vi "Read AIP Status.vi"(8 "error in (no error)":errorcluster, 11 "AIP Status Response in":refnum<class "AIP Status Response.lvclass">) -> (0 "error out":errorcluster, 1 "AIP Depth Min":u8, 2 "AIP Status":T1, 3 "AIP Status Response out":refnum<class "AIP Status Response.lvclass">)   [LabVIEW 2015, in "RDS Child Messages.lvlib" / "AIP Status Response.lvclass"]
uses:
  AIP Status Response.lvclass
  RDS Instruments/AIP/AIP Status.ctl
  RDS Instruments/AIP/AIP States.ctl
  RDS Serial Handler/RDS Serial Frame.lvclass
  AIP Status Response.lvclass/AIP Status Response.ctl
  RDS Instruments/RDS Instrument Library.lvlib
panel:
  out "Raw Frame":refnum<class "RDS Serial Frame.lvclass">
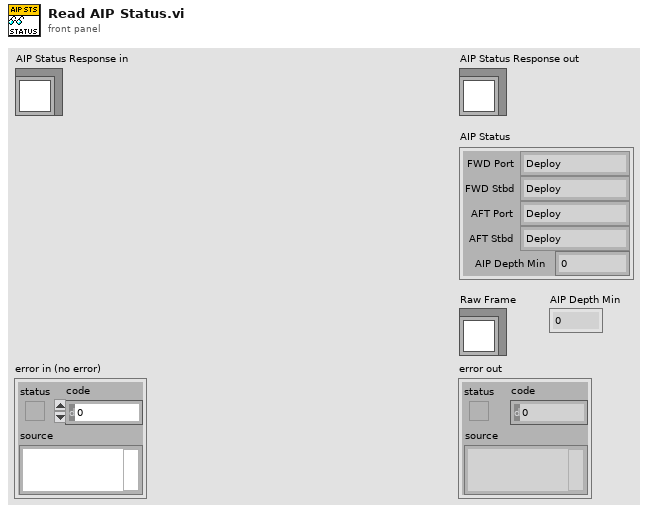
[diagram p1: front panel]
types:
  T1 = typedef "RDS Instrument Library.lvlib/AIP Status.ctl" = cluster{"FWD Port":T2, "FWD Stbd":T2, "AFT Port":T2, "AFT Stbd":T2, "AIP Depth Min":u8}
  T2 = typedef "RDS Instrument Library.lvlib/AIP States.ctl" = enum16{"Deploy", "Deploying", "Deployed", "Stow", "Stowing", "Stowed", "Fault", "brakeOnStow", "breakOnDeploy", "Stopped", "Stopping"}
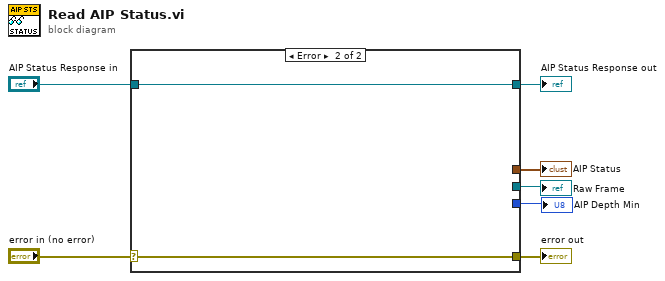
[diagram p0: block diagram]
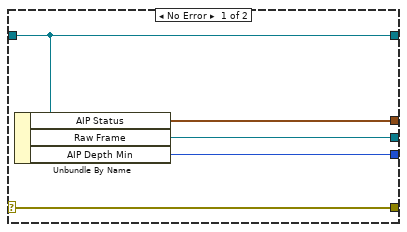
[diagram p2: hidden frame]
diagram:
  n1 = case shown="Error" "error in (no error)" {
    selector: "error in (no error)" -> [w12 w13]
    tunnel: [w12 w13] -> w6
    tunnel: [w11 w14] -> w4
    tunnel: "AIP Status Response in" -> [w11 w14]
    tunnel: [w10 _] -> w3
    tunnel: [w9 _] -> w2
    tunnel: [w8 _] -> w1
    frame No Error {
      n2 = Unbundle By Name(w11) -> ("AIP Status"=w10:T1, "Raw Frame"=w9:refnum<class "RDS Serial Frame.lvclass">, "AIP Depth Min"=w8:u8)
    }
    frame Error {
    }
  }
  "error out" <- w6
  "AIP Status Response out" <- w4
  "AIP Status" <- w3
  "Raw Frame" <- w2
  "AIP Depth Min" <- w1
